vi "DI_Read.vi"(8 "error in (no error)":errorcluster, 9 "Stop DI":bool, 11 "reference in":refnum<class "DI.lvclass">) -> (0 "error out":errorcluster, 3 "reference out":refnum<class "DI.lvclass">)   [LabVIEW 2017, in "DI.lvclass"]
uses:
  DI.lvclass
panel:
  # "This VI is called Asynchronously and will have one instance in memory\nfor each asynchronous call."
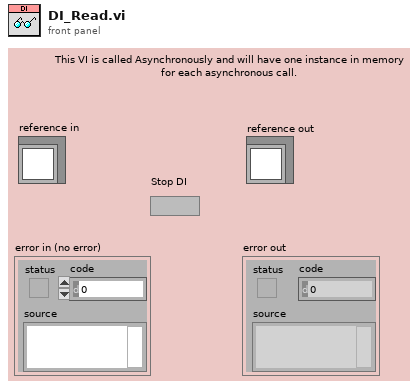
[diagram p1: front panel]
types:
  T1 = typedef "DI.lvclass/ObjectAttributes.ctl" = cluster{"DI Task":refnum<k21>, "DI Status":bool[], "DI Module Names (NI-Max Name)":string[], "Number of Channels Per DI Module":i32[], "Number of DI Modules":u32, "Number of Total DI Channels":u32, "DI On/Off Status":bool, "DO VI Reference":refnum<vi>}
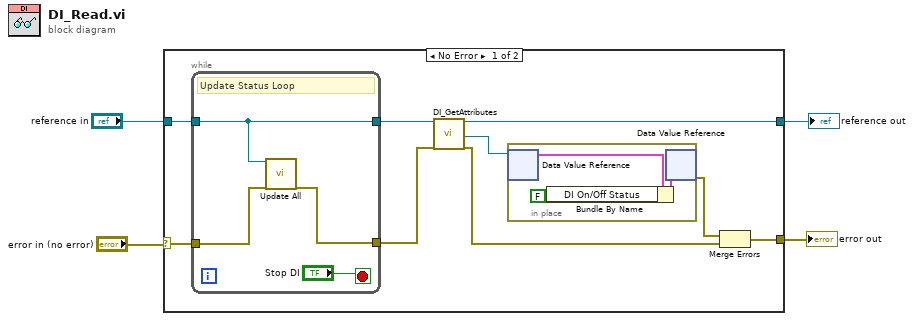
[diagram p0: block diagram]
diagram:
  n1 = case shown="No Error" "error in (no error)" {
    selector: "error in (no error)" -> [w13 w22]
    tunnel: "reference in" -> [w12 w21]
    tunnel: [w6 w21] -> w2
    tunnel: [w5 w22] -> w1
    frame No Error {
      n2 = while {
        tunnel: [w14] -> w9
        tunnel: w13 -> [w15]
        tunnel: w12 -> [w16]
        tunnel: [w16] -> w10
        stop <- "Stop DI" stop-if-true
        # "Update Status Loop"
        n3 = call-dynamic "Update All.vi"("reference in"=w16, "error in (no error)"=w15) -> ("error out"=w14:errorcluster)  [unwired: 16 in, 1 out]
      }
      n4 = call "DI_GetAttributes.vi"("reference in"=w10, "error in (no error)"=w9) -> ("reference out"=w6:refnum<class "DI.lvclass">, "DataRef"=w7:refnum<data-value>, "error out"=w8:errorcluster)  [unwired: 14 in, 1 out]
      n5 = in-place {
        n6 = in-place-dvr #1(w7) -> (w20:T1)  [unwired: 1 out]
        n7 = Bundle By Name(cluster=w20, "DI On/Off Status"=FALSE) -> (w19:T1)
        n8 = in-place-dvr #1(w19) -> (w11:errorcluster)  [unwired: 1 out]
      }
      n9 = Merge Errors(w11, w8) -> (w5:errorcluster)
    }
    frame Error {
    }
  }
  "reference out" <- w2
  "error out" <- w1
